vi "Choreo_TrajectoryState_Flipped.vi"(11 "ChoreoTrajectoryState":T1) -> (3 "flipped ChoreoTrajectoryState":T1)   [LabVIEW 2019]
doc: "Return \"flipped:\" trajectory state, mirrored accros the field mid-line.\n\nInputs:\n - ChoreoTrajectoryState - cluster - Individual trajectory state\n\nOutputs: \n - Flipped_ChoreoTrajectoryState - cluster -this state, mirrored across the field midline."
uses:
  TypeDef/ChoreoTrajectoryState.ctl
  ChoreoLib.lvlib
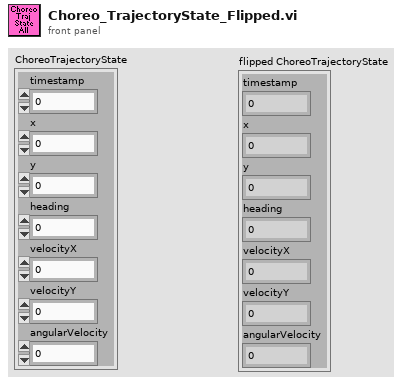
[diagram p1: front panel]
types:
  T1 = typedef "ChoreoLib.lvlib/ChoreoTrajectoryState.ctl" = cluster{"timestamp":dbl, "x":dbl, "y":dbl, "heading":dbl, "velocityX":dbl, "velocityY":dbl, "angularVelocity":dbl}
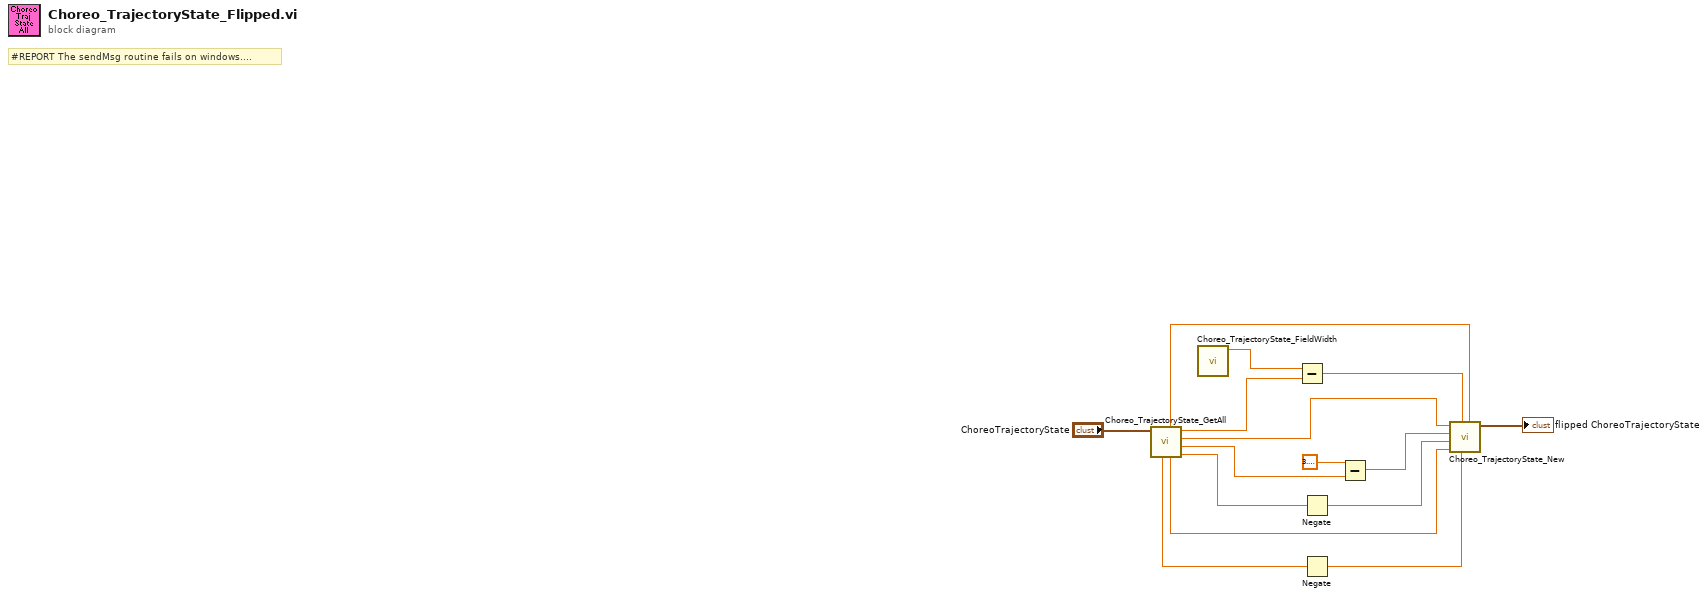
[diagram p0: block diagram]
diagram:
  # "#REPORT The sendMsg routine fails on windows...."
  n1 = call "Choreo_TrajectoryState_GetAll.vi"("ChoreoTrajectoryState"="ChoreoTrajectoryState") -> ("velocityX"=w5:dbl, "heading"=w8:dbl, "y"=w9:dbl, "x"=w12:dbl, "velocityY"=w3:dbl, "timestamp"=w13:dbl, "angularVelocity"=w2:dbl)  [unwired: 4 in]
  n2 = call "Choreo_TrajectoryState_FieldWidth.vi"() -> ("Field_Width_Meters"=w11:dbl)  [unwired: 11 in]
  n3 = Subtract(x=w11, y=w12) -> (x-y=w10:dbl)
  n4 = Negate(x=w5) -> (-x=w4:dbl)
  n5 = Negate(x=w2) -> (-x=w1:dbl)
  n6 = Subtract(x=3.141592653589793, y=w8) -> (x-y=w7:dbl)
  n7 = call "Choreo_TrajectoryState_New.vi"("timestamp"=w13, "angularVelocity"=w1, "x"=w10, "velocityY"=w3, "velocityX"=w4, "heading"=w7, "y"=w9) -> ("ChoreoTrajectoryState"=→"flipped ChoreoTrajectoryState":T1)  [unwired: 4 in]
